vi "Read Holding Registers.vi"(8 "error in (no error)":errorcluster, 9 "number of holding registers":u16, 10 "starting address":u16, 11 "Modbus slave in":refnum<class "Modbus Master CR API.lvclass">) -> (0 "error out":errorcluster, 2 "register values":u16[](array[numeric]), 3 "Modbus slave out":refnum<class "Modbus Master CR API.lvclass">)   [LabVIEW 2021, in "Modbus Master CR API.lvclass"]
doc: "Reads values of contiguous holding registers."
uses:
  Modbus Master CR API.lvclass
  Modbus Master CR API.lvclass/Modbus Master CR API.ctl
  Data Model/Device Data Model.lvclass
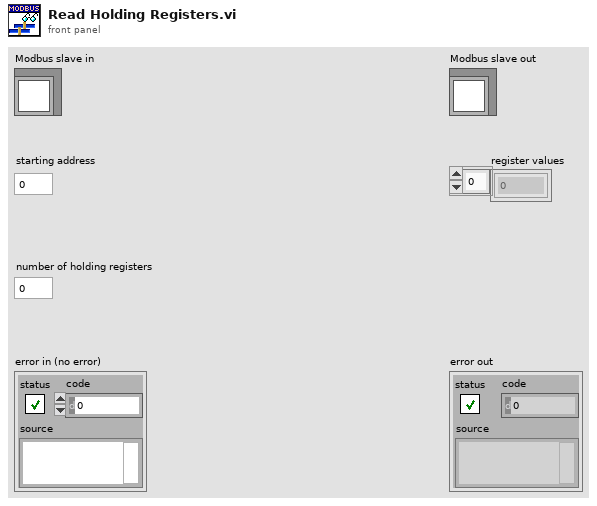
[diagram p1: front panel]
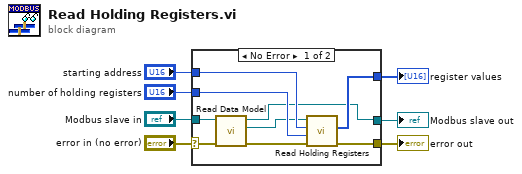
[diagram p0: block diagram]
diagram:
  n1 = case shown="No Error" "error in (no error)" {
    selector: "error in (no error)" -> [w12 w17]
    tunnel: [w16 w17] -> w7
    tunnel: [w8 w18] -> w6
    tunnel: [w15 _] -> w5
    tunnel: "Modbus slave in" -> [w9 w18]
    tunnel: "starting address" -> [w14 _]
    tunnel: "number of holding registers" -> [w13 _]
    frame No Error {
      n2 = call "Read Data Model.vi"("error in (no error)"=w12, "Modbus slave in"=w9) -> ("error out"=w11:errorcluster, "device data model"=w10:refnum<class "Device Data Model.lvclass">, "Modbus slave out"=w8:refnum<class "Modbus Master CR API.lvclass">)  [unwired: 7 in]
      n3 = call-dynamic "Read Holding Registers.vi"("error in"=w11, "number of registers"=w13, "starting address"=w14, "device data model in"=w10) -> ("error out"=w16:errorcluster, "data"=w15:u16[])  [unwired: 5 in, 1 out]
    }
    frame Error {
    }
  }
  "error out" <- w7
  "Modbus slave out" <- w6
  "register values" <- w5
